vi "data_base_mt_connect_3 (SubVI).vi"(0 "Byte Stream File in":refnum<file>, 1 "base path":path, 2 "G1?":u32, 4 "Machine type":string, 5 "error in (no error)":errorcluster, 8 "Machine parameters":string[](array[string]), 10 "data":dbl[](array[numeric]), 12 "current time":timestamp, 18 "Machine Data 2":T1) -> (14 "Byte Stream File out":refnum<file>, 19 "error out":errorcluster)   [LabVIEW 2014]
panel:
  out "First Call?: T/F":bool
  out "appended path 2":path
  out "error out 2":errorcluster
  in  "error in (no error) 2":errorcluster
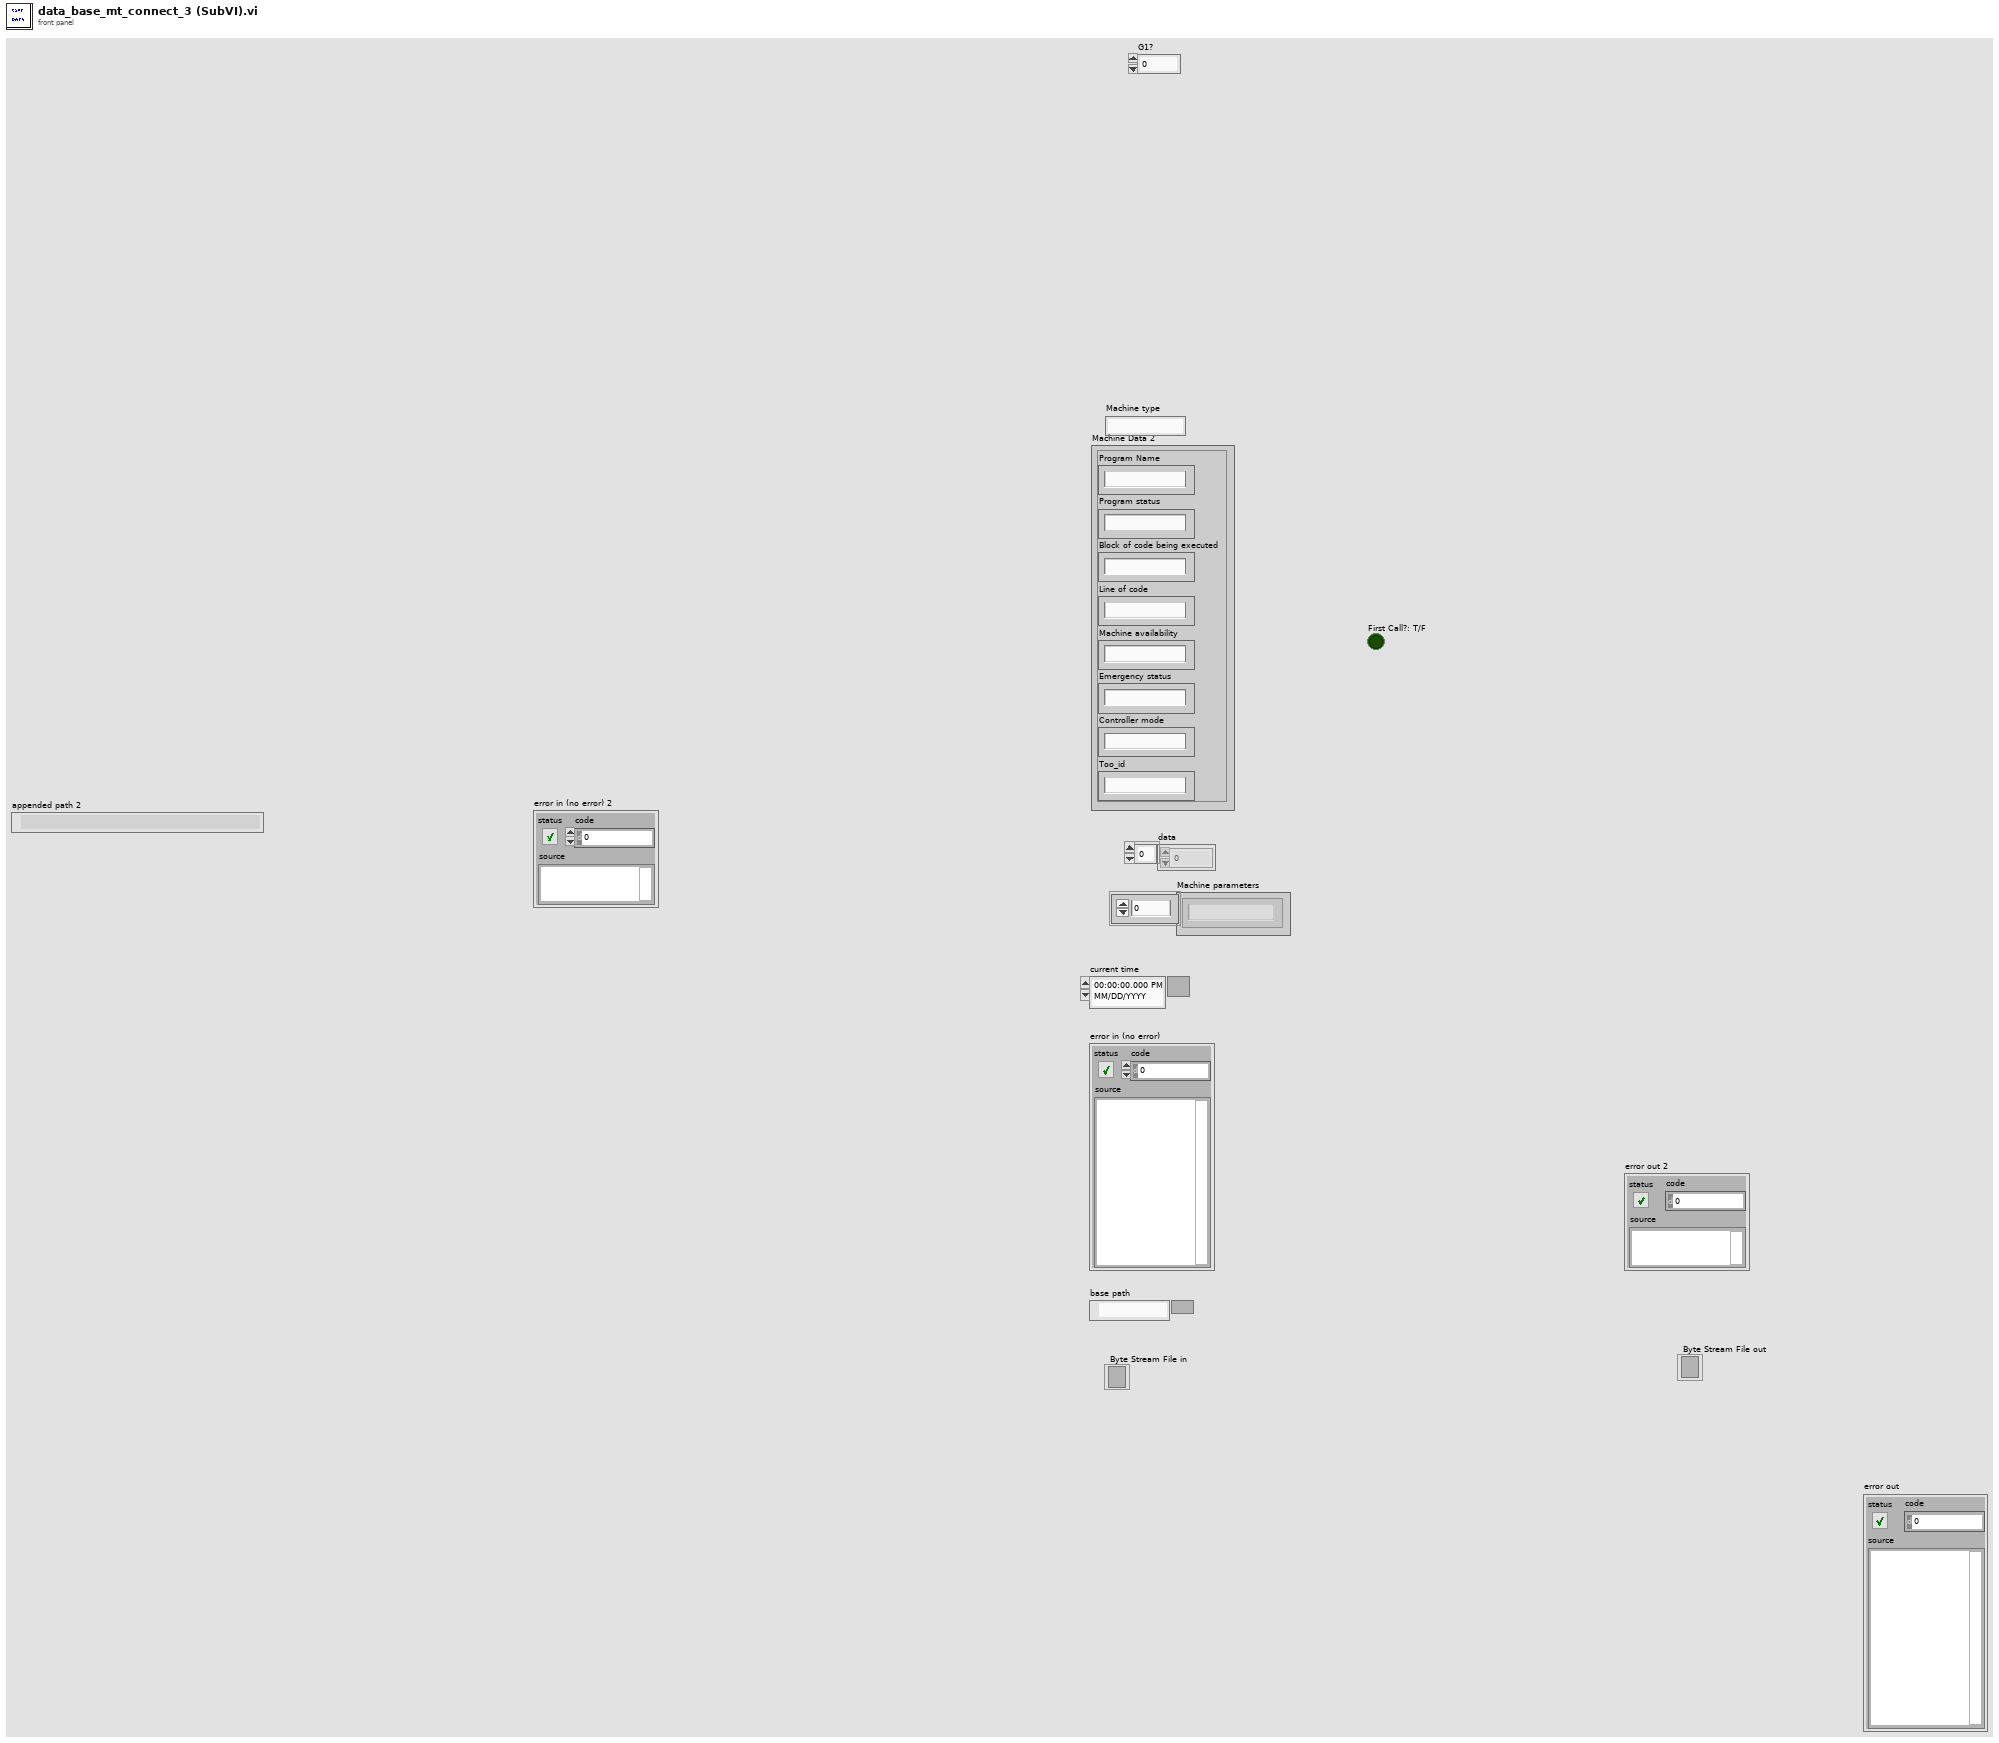
[diagram p1: front panel]
types:
  T1 = cluster{"Program Name":string, "Program status":string, "Block of code being executed":string, "Line of code":string, "Machine availability":string, "Emergency status":string, "Controller mode":string, "Too_id":string}
  T2 = enum16{"open", "replace", "create", "open or create", "replace or create", "replace or create with confirmation"}
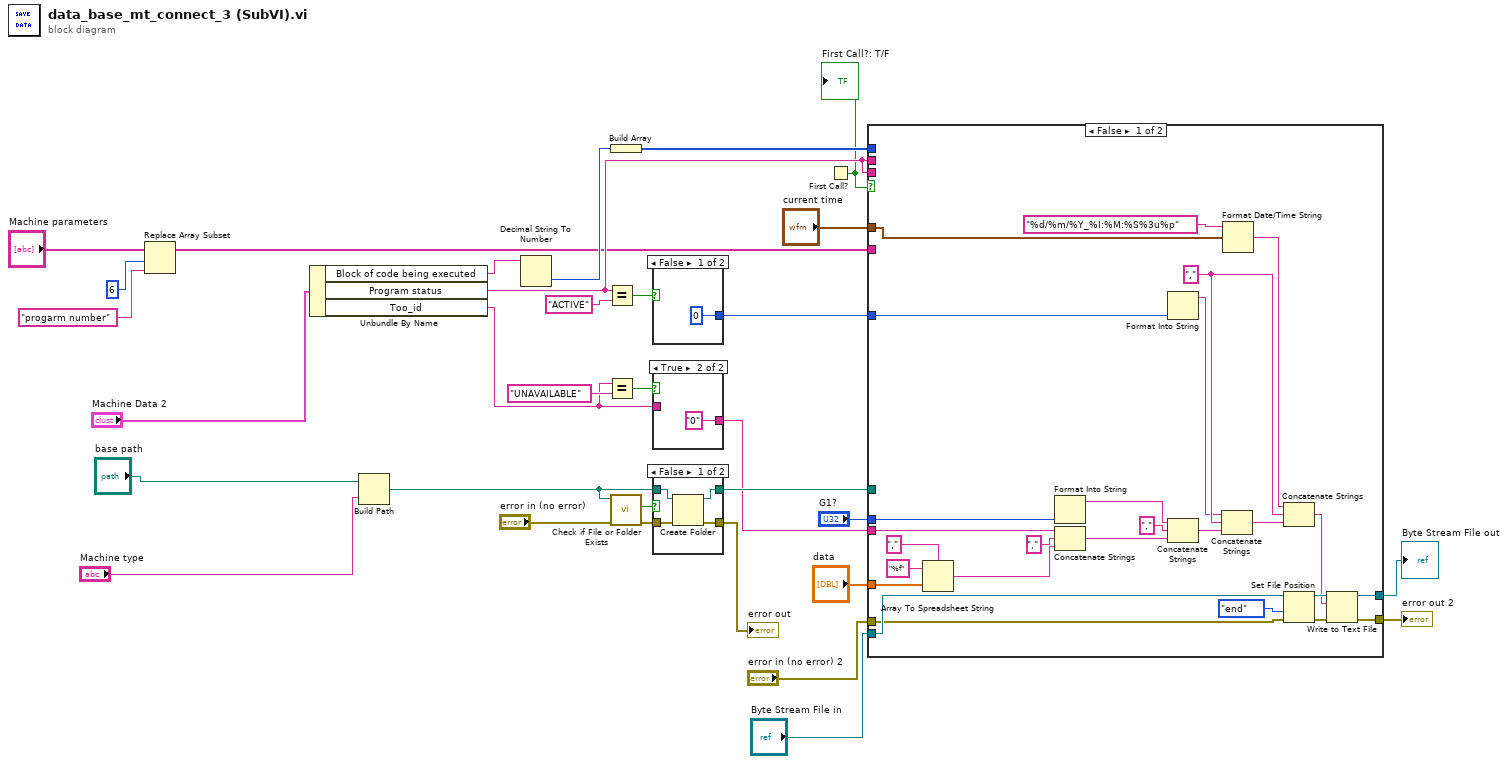
[diagram p0: block diagram]
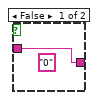
[diagram p2: hidden frame]
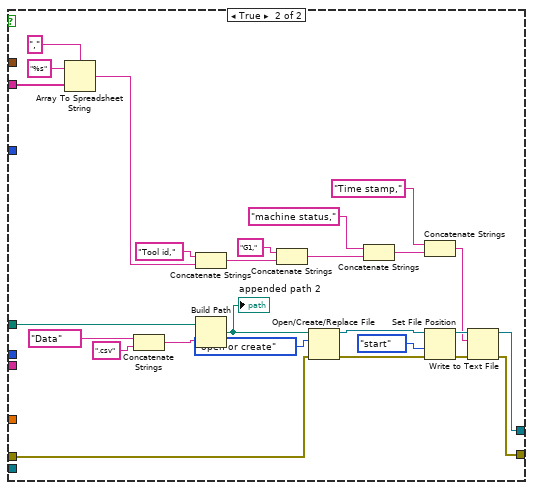
[diagram p3: hidden frame]
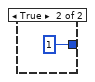
[diagram p4: hidden frame]
diagram:
  n1 = Replace Array Subset(array="Machine parameters", new element="progarm number" ("new element/subarray"), index=6) -> (w2:string[])
  n2 = Unbundle By Name("Machine Data 2") -> ("Block of code being executed"=w17:string, "Program status"=w16:string, "Too_id"=w4:string)
  n3 = Build Path(base path="base path", name or relative path="Machine type") -> (appended path=w14:path)
  n4 = Decimal String To Number(string=w17) -> (number=w18:i32)  [unwired: 2 in, 1 out]
  n5 = Equal?(x=w16, y="ACTIVE") -> (x = y?=w9:bool)
  n6 = Equal?(x=w4, y="UNAVAILABLE") -> (x = y?=w5:bool)
  n7 = Build Array(w18) -> (w19:i32[])
  n8 = call <vilib>:"Check if File or Folder Exists.vi"("error in (no error)"="error in (no error)", "path"=w14) -> ("error out"=w28:errorcluster, "file or folder exists?"=w29:bool)  [unwired: 7 in, 1 out]
  n9 = case shown="False" w9 {
    tunnel: [0 1] -> w8
    frame False {
    }
    frame True {
    }
  }
  n10 = case shown="True" w5 {
    tunnel: w4 -> [w35 _]
    tunnel: [w35 "0"] -> w3
    frame False {
      (unwired) "0"
    }
    frame True {
    }
  }
  n11 = case shown="False" w29 {
    tunnel: [w40 w42] -> w30
    tunnel: w28 -> [w39 w42]
    tunnel: w14 -> [w38 w41]
    tunnel: [w37 w41] -> w25
    frame False {
      n12 = Create Folder(path (use dialog)=w38, error in=w39) -> (created path=w37:path, error out=w40:errorcluster)  [unwired: 1 in, 1 out]
    }
    frame True {
    }
  }
  "error out" <- w30
  n13 = First Call?() -> (First Call?: T/F=w7:bool)
  "First Call?: T/F" <- w7
  n14 = case shown="False" w7 {
    tunnel: w25 -> [_ w79]
    tunnel: "error in (no error) 2" -> [w58 w70]
    tunnel: [w57 w76] -> w27
    tunnel: [w60 w78] -> w24
    tunnel: "Byte Stream File in" -> [w59 _]
    tunnel: "current time" -> [w56 _]
    tunnel: "G1?" -> [w61 _]
    tunnel: "data" -> [w55 _]
    tunnel: w2 -> [_ w77]
    tunnel: w19 -> [_ _]
    tunnel: w16 -> [_ _]
    tunnel: w16 -> [_ _]
    tunnel: w3 -> [w46 _]
    tunnel: w8 -> [w44 _]
    frame False {
      w48 = "," ("string")
      n15 = Array To Spreadsheet String(delimiter (Tab)=",", array=w55, 3:"%f" ("format string")) -> (spreadsheet string=w51:string)
      n16 = Format Into String(w61) -> (resulting string=w63:string)  [unwired: 3 in, 1 out]
      n17 = Concatenate Strings(w46, "," ("string"), w51) -> (w62:string)
      n18 = Format Into String(w44) -> (resulting string=w43:string)  [unwired: 3 in, 1 out]
      n19 = Concatenate Strings(w63, "," ("string"), w62) -> (w50:string)
      n20 = Concatenate Strings(w43, w48, w50) -> (w49:string)
      n21 = Format Date/Time String(time format string (%c)="%d/%m/%Y_%I:%M:%S%3u%p", seconds (now)=w56) -> (date/time string=w45:string)  [unwired: 1 in]
      n22 = Concatenate Strings(w45, w48, w49) -> (w47:string)
      n23 = Set File Position(refnum=w59, from (0:start)=enum16{"start", "end", "current"}."end", error in=w58) -> (refnum out=w67:refnum<file>, error out=w66:errorcluster)  [unwired: 1 in]
      n24 = Write to Text File(file (use dialog)=w67, text=w47, error in=w66) -> (refnum out=w60:refnum<file>, error out=w57:errorcluster)  [unwired: 1 in, 1 out]
    }
    frame True {
      n25 = Array To Spreadsheet String(delimiter (Tab)=",", array=w77, 3:"%s" ("format string")) -> (spreadsheet string=w84:string)
      n26 = Concatenate Strings("Data" ("string"), ".csv" ("string")) -> (w94:string)
      n27 = Concatenate Strings("Tool id," ("string"), w84) -> (w81:string)
      n28 = Build Path(base path=w79, name or relative path=w94) -> (appended path=w83:path)
      "appended path 2" <- w83
      n29 = Concatenate Strings("G1," ("string"), w81) -> (w74:string)
      n30 = Open/Create/Replace File(file path (use dialog)=w83, error in=w70, operation (0:open)=T2."open or create") -> (refnum out=w92:refnum<file>, error out=w91:errorcluster)  [unwired: 3 in, 1 out]
      n31 = Concatenate Strings("machine status," ("string"), w74) -> (w73:string)
      n32 = Concatenate Strings("Time stamp," ("string"), w73) -> (w71:string)
      n33 = Set File Position(refnum=w92, from (0:start)=enum16{"start", "end", "current"}."start", error in=w91) -> (refnum out=w88:refnum<file>, error out=w89:errorcluster)  [unwired: 1 in]
      n34 = Write to Text File(file (use dialog)=w88, text=w71, error in=w89) -> (refnum out=w78:refnum<file>, error out=w76:errorcluster)  [unwired: 1 in, 1 out]
    }
  }
  "Byte Stream File out" <- w24
  "error out 2" <- w27
